vi "6.5test.vi"() -> ()   [LabVIEW 2018]
uses:
  <vilib>/Instr/_visa.llb/VISA Configure Serial Port (Instr).vi
panel:
  in  "TCP HEX":bool
  in  "设置端口号":string
  in  "创建8266服务器":bool
  in  "字符串3":string
  in  "确定按钮3":bool
  in  "字符串2":string
  in  "确定按钮2":bool
  in  "字符串1":string
  in  "确定按钮1":bool
  in  "多条串口发送":bool
  in  "确定按钮0":bool
  in  "字符串0":string
  in  "清空TCP内容":bool
  in  "TCP发送消息框":string
  in  "TCP发送":bool
  in  "服务器发送":bool
  in  "远程端口":u16
  in  "远程IP":string
  in  "开启监听":bool
  in  "查看当前建立连接":bool
  out "TCP接收信息框":string
  in  "自动添加回车":bool
  in  "十六进制发送":bool
  in  "串口HEX":bool
  in  "清空数据":bool
  in  "IP按钮":bool
  in  "WIFI密码":string
  in  "WIFI用户名":string
  in  "连入wifi":bool
  in  "重启按钮":bool
  in  "AT测试按钮":bool
  in  "停止":bool
  out "串口接收信息框":string
  in  "串口发送":bool
  in  "串口发送消息框":string
  in  "baud rate (9600)":u32=9600 caption="波特率"
  in  "VISA resource name":refnum<visa-resource-name> caption="串口号"
  # "串口配置"
  # "TCP CLIENT配置"
  # "ESP8266 功能选择"
  # "串口信息"
  # "TCP CLIENT信息"
  # "多条串口发送 / AT指令"
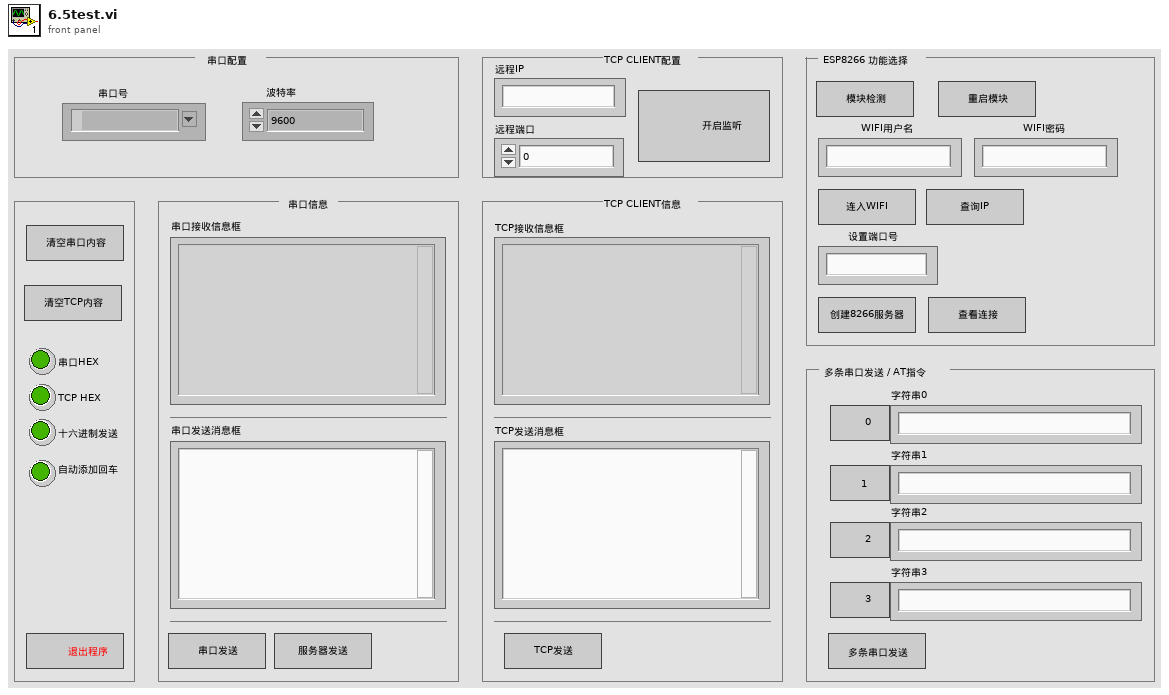
[diagram p1: front panel]
types:
  T1 = enum16{"Standard", "Buffered", "CRLF", "Immediate"}
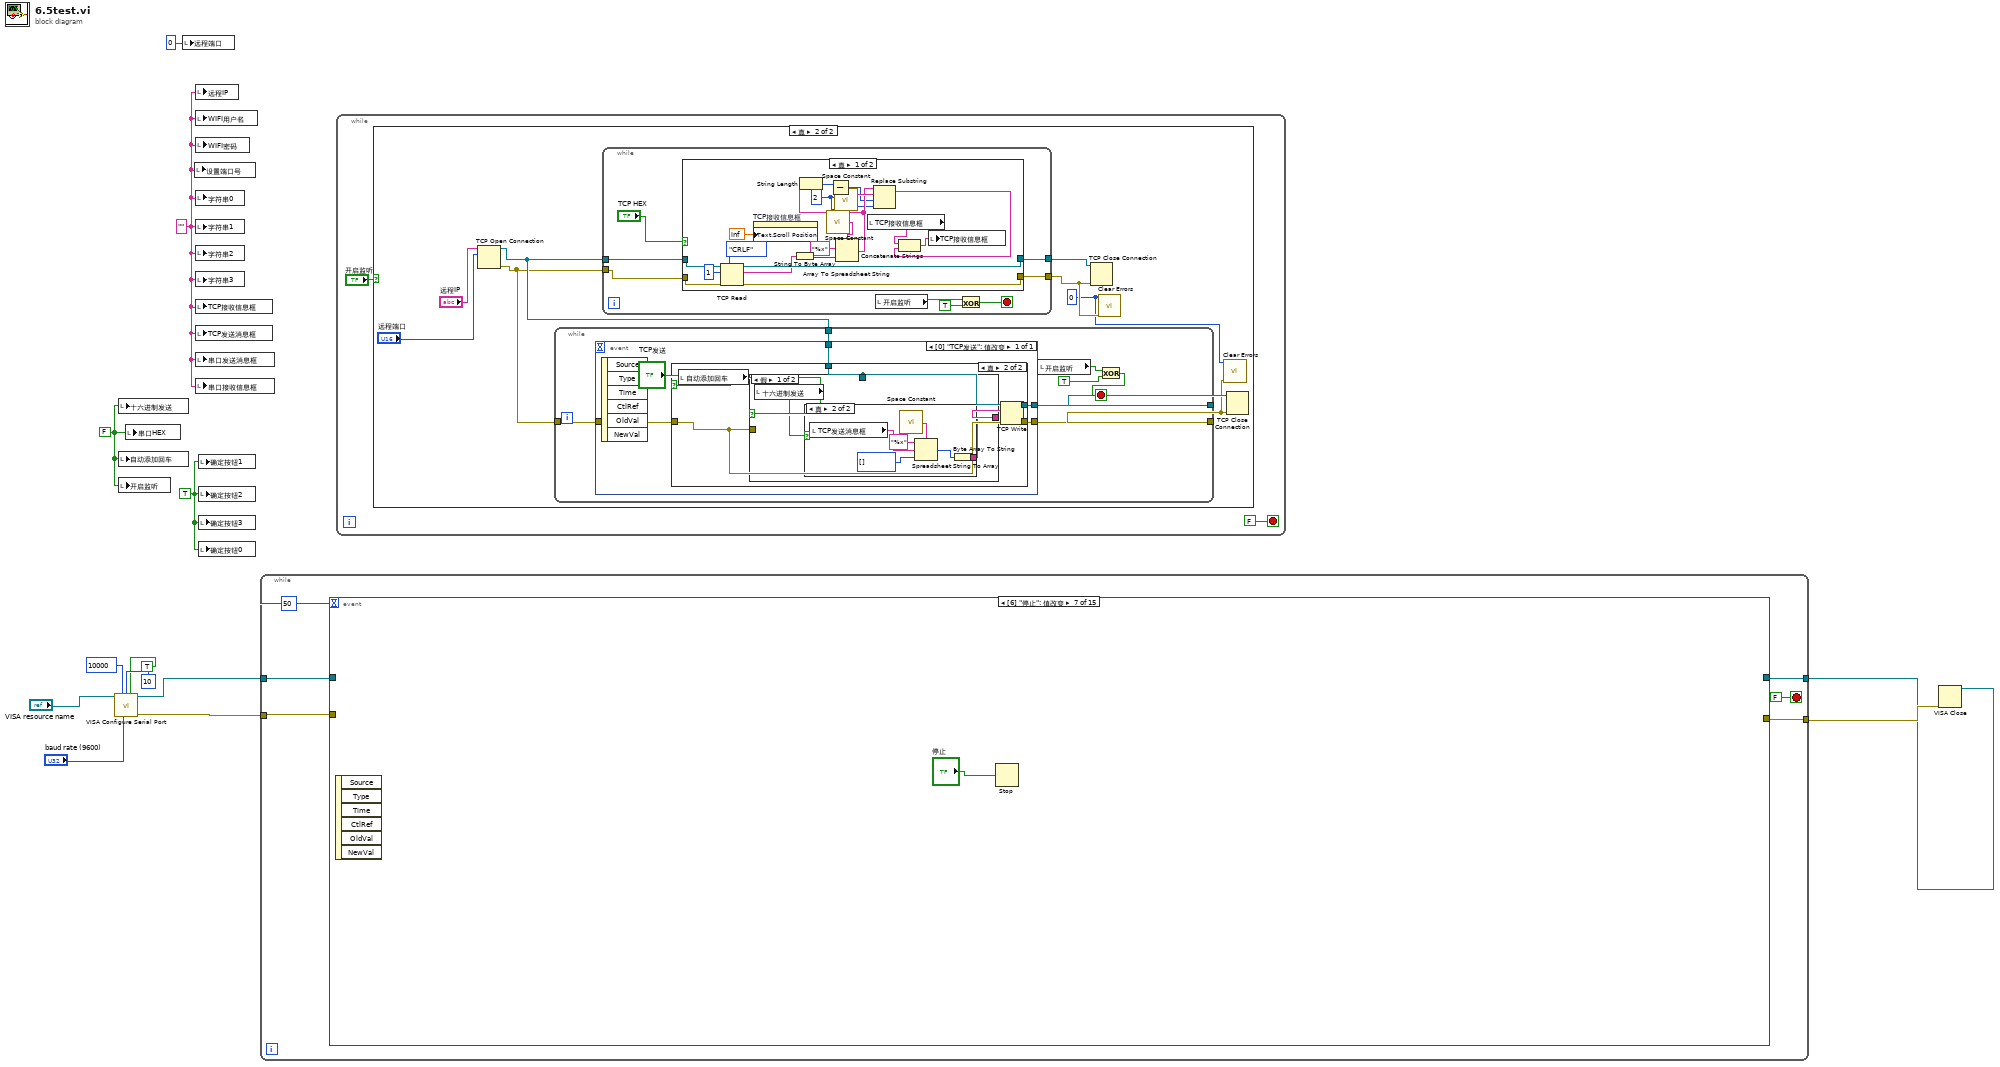
[diagram p0: block diagram]
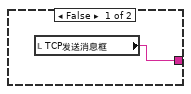
[diagram p4: hidden frame]
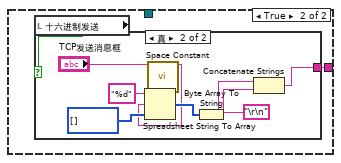
[diagram p5: hidden frame]
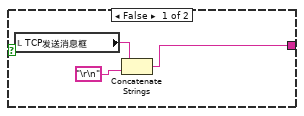
[diagram p6: hidden frame]
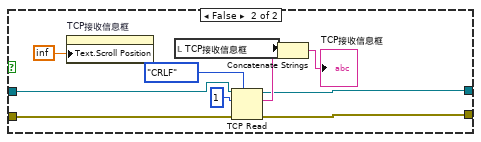
[diagram p7: hidden frame]
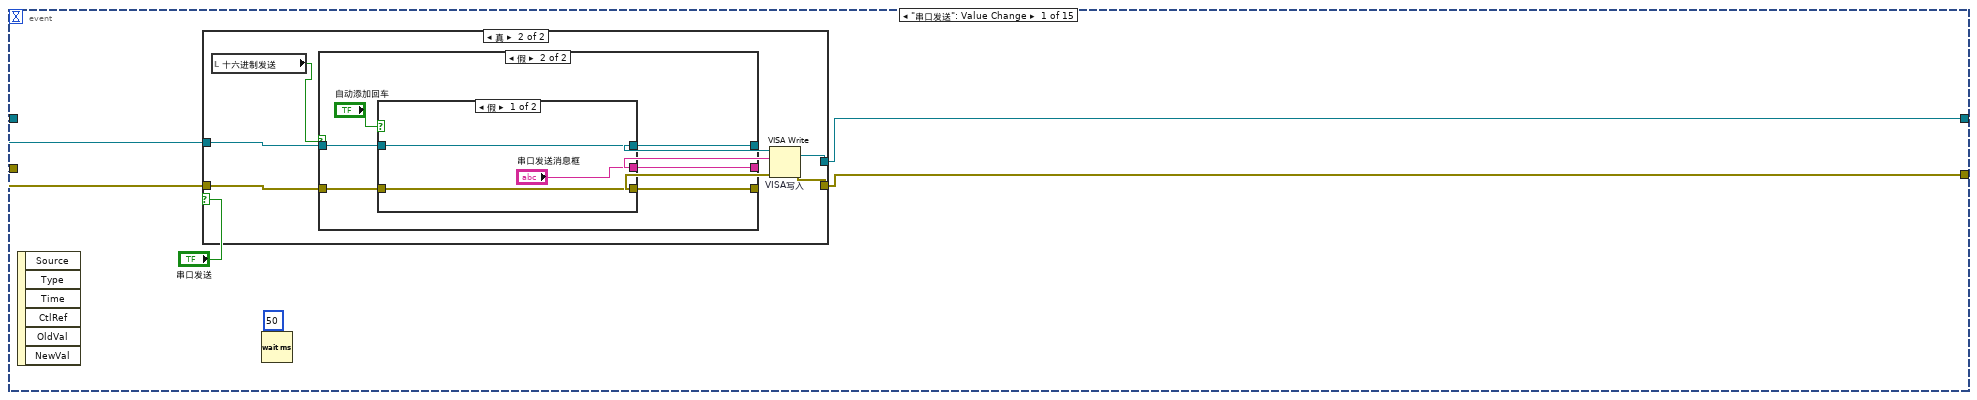
[diagram p8: hidden frame]
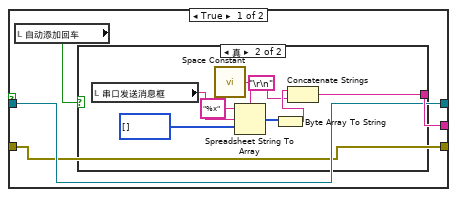
[diagram p10: hidden frame]
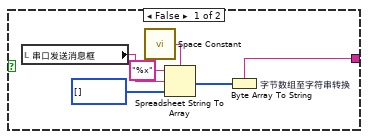
[diagram p11: hidden frame]
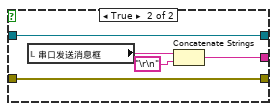
[diagram p12: hidden frame]
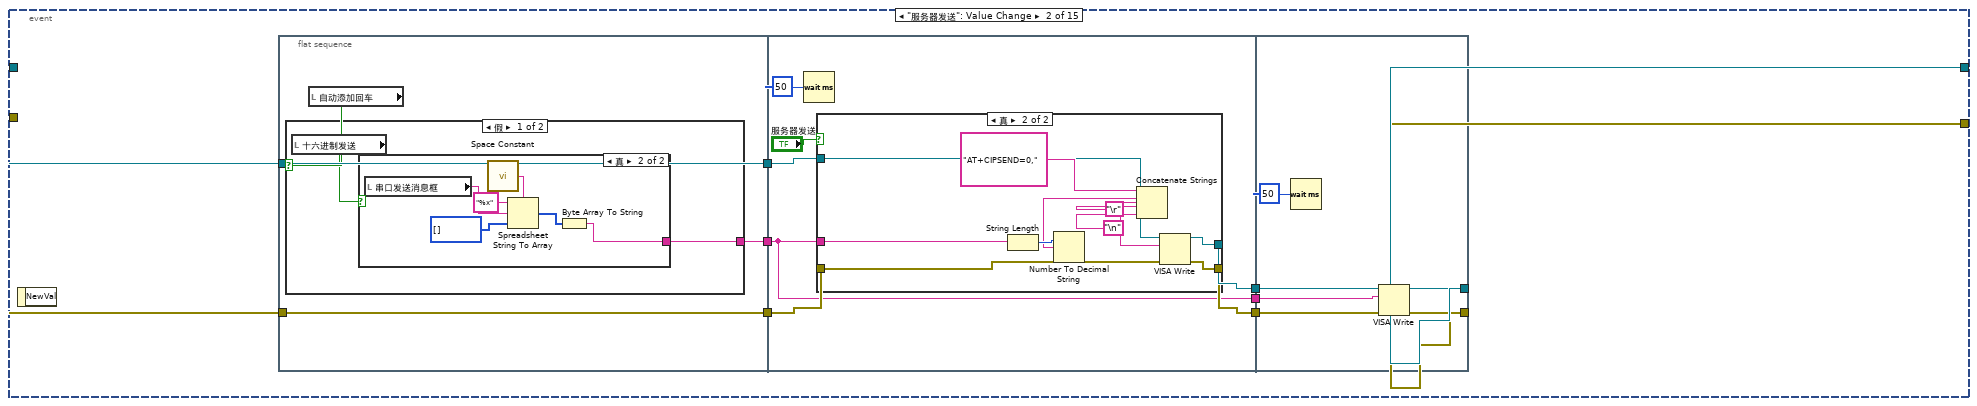
[diagram p13: hidden frame]
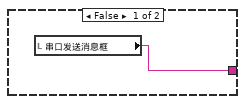
[diagram p14: hidden frame]
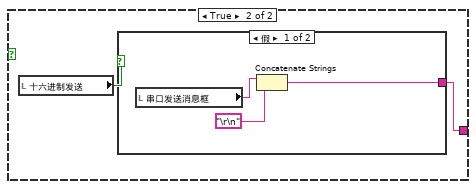
[diagram p15: hidden frame]
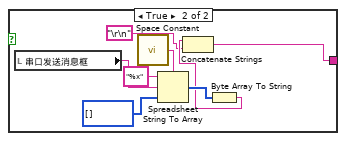
[diagram p16: hidden frame]
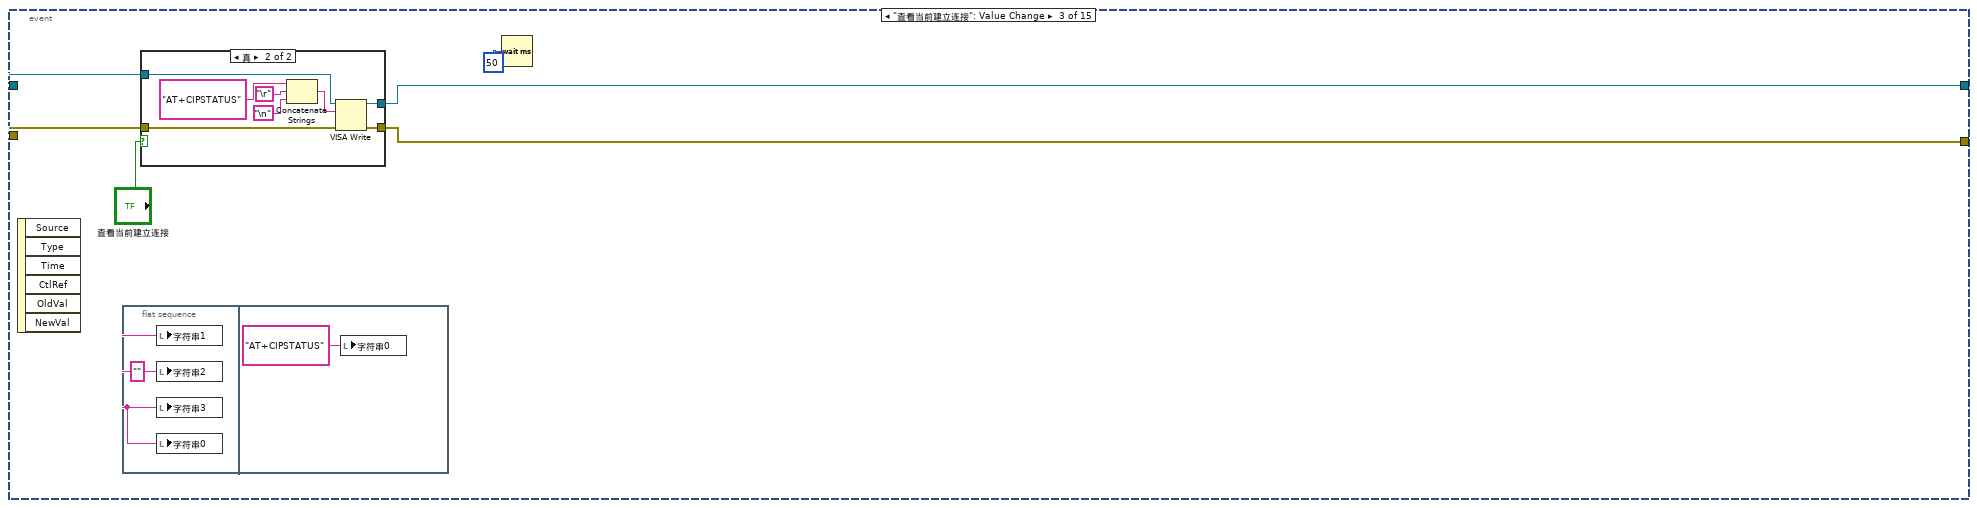
[diagram p18: hidden frame]
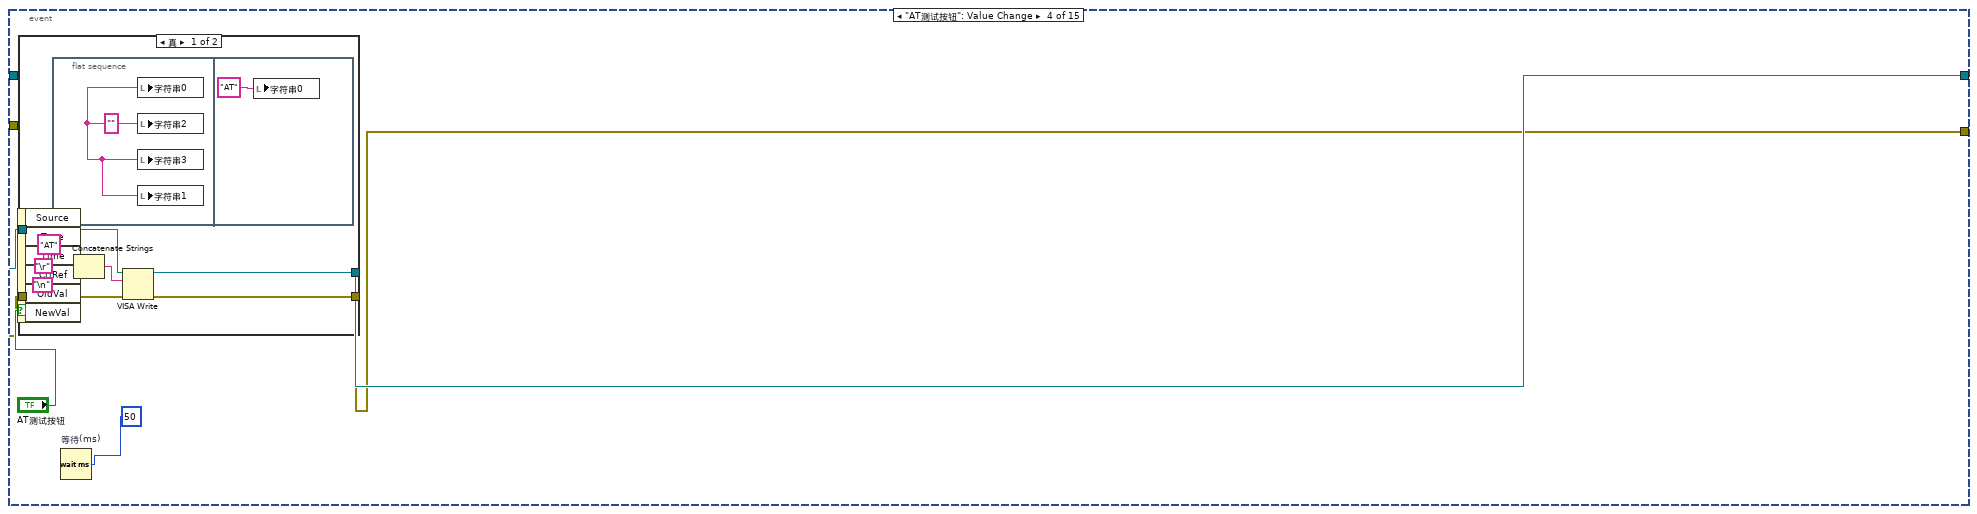
[diagram p20: hidden frame]
diagram:
  w1 = FALSE ("开启监听")
  w2 = "" ("字符串2")
  w4 = TRUE ("确定按钮0")
  n1 = call-poly "VISA Configure Serial Port"("VISA resource name"="VISA resource name", "timeout (10sec)"=u32 10000, "termination char\n(0xA = '\\n' = LF)"=u8 10 ("termination char\n(0xA = '\\n' = LF)"), "Enable Termination\nChar (T)"=TRUE ("Enable Termination\nChar (T)"), "baud rate (9600)"="baud rate (9600)") -> ("VISA resource name out"=w7:refnum<visa-resource-name>, "error out"=w6:errorcluster)  [unwired: 9 in]
  n2 = local write "十六进制发送"(w1) -> ()
  n3 = local write "自动添加回车"(w1) -> ()
  n4 = local write "开启监听"(w1) -> ()
  n5 = local write "串口HEX"(w1) -> ()
  n6 = local write "远程端口"(u16 0 ("远程端口")) -> ()
  n7 = local write "设置端口号"(w2) -> ()
  n8 = local write "远程IP"(w2) -> ()
  n9 = local write "WIFI用户名"(w2) -> ()
  n10 = local write "WIFI密码"(w2) -> ()
  n11 = local write "字符串0"(w2) -> ()
  n12 = local write "字符串1"(w2) -> ()
  n13 = local write "字符串2"(w2) -> ()
  n14 = local write "字符串3"(w2) -> ()
  n15 = local write "TCP接收信息框"(w2) -> ()
  n16 = local write "TCP发送消息框"(w2) -> ()
  n17 = local write "串口发送消息框"(w2) -> ()
  n18 = local write "串口接收信息框"(w2) -> ()
  n19 = local write "确定按钮1"(w4) -> ()
  n20 = local write "确定按钮2"(w4) -> ()
  n21 = local write "确定按钮3"(w4) -> ()
  n22 = local write "确定按钮0"(w4) -> ()
  n23 = while {
    tunnel: w6 -> [w18]
    tunnel: w7 -> [w19]
    tunnel: [w15] -> w5
    tunnel: [w14] -> w8
    stop <- FALSE stop-if-true
    n24 = event shown="[6] \"停止\": 值改变" {
      selector: _ -> [_ _ _ _ _ _ _ _ _ _ _ _ _ _ _]
      dyn-events: _ -> [_ _ _ _ _ _ _ _ _ _ _ _ _ _ _]
      timeout: 50 -> [_ _ _ _ _ _ _ _ _ _ _ _ _ _ _]
      tunnel: w19 -> [w24 w77 w132 w148 w172 w197 _ w214 w237 w301 w388 _ _ _ _]
      tunnel: w18 -> [w23 w76 w131 w147 w171 w196 _ w213 w236 w300 w387 _ _ _ _]
      tunnel: [w22 w73 w130 w146 w170 w195 _ w212 w235 w298 w386 _ _ _ _] -> w15
      tunnel: [w21 w72 w129 w145 w169 w194 _ w211 w234 w299 w385 _ _ _ _] -> w14
      event "串口发送": Value Change {
        n25 = event-data() -> ()  [unwired: 1 in, 6 out]
        n26 = case shown="真" "串口发送" {
          tunnel: w24 -> [w27 w35]
          tunnel: w23 -> [w26 w34]
          tunnel: [w27 w31] -> w22
          tunnel: [w26 w32] -> w21
          frame False {
          }
          frame True {
            n27 = local read "十六进制发送"() -> (w28:bool)
            n28 = case shown="假" w28 {
              tunnel: w35 -> [w38 w59]
              tunnel: w34 -> [w37 w58]
              tunnel: [w39 w57] -> w33
              tunnel: [w38 w55] -> w30
              tunnel: [w37 w54] -> w29
              frame True {
                n29 = local read "自动添加回车"() -> (w36:bool)
                n30 = case shown="真" w36 {
                  tunnel: [w40 w47] -> w39
                  frame False {
                    n31 = local read "串口发送消息框"() -> (w44:string)
                    n32 = call <vilib>:"Space Constant.vi"() -> ("String"=w45:string)
                    n33 = Spreadsheet String To Array(delimiter (Tab)=w45, format string="%x" ("格式字符串"), spreadsheet string=w44, array type (2D Dbl)=u8[] []) -> (array=w41:u8[])
                    n34 = Byte Array To String "字节数组至字符串转换"(unsigned byte array=w41) -> (string=w40:string)
                  }
                  frame True {
                    n35 = local read "串口发送消息框"() -> (w51:string)
                    n36 = call <vilib>:"Space Constant.vi"() -> ("String"=w52:string)
                    n37 = Spreadsheet String To Array(delimiter (Tab)=w52, format string="%x" ("格式字符串"), spreadsheet string=w51, array type (2D Dbl)=u8[] []) -> (array=w53:u8[])
                    n38 = Byte Array To String(unsigned byte array=w53) -> (string=w48:string)
                    n39 = Concatenate Strings(w48, "\r\n") -> (w47:string)
                  }
                }
              }
              frame False {
                n40 = case shown="假" "自动添加回车" {
                  tunnel: w59 -> [w61 w66]
                  tunnel: w58 -> [w60 w65]
                  tunnel: ["串口发送消息框" w67] -> w57
                  tunnel: [w61 w66] -> w55
                  tunnel: [w60 w65] -> w54
                  frame False {
                  }
                  frame True {
                    n41 = local read "串口发送消息框"() -> (w63:string)
                    n42 = Concatenate Strings ("连接字符串")(w63, "\r\n") -> (w67:string)
                  }
                }
              }
            }
            n43 = VISA Write "VISA写入"(VISA resource name=w30, write buffer=w33, error in (no error)=w29) -> (VISA resource name out=w31:refnum<visa-resource-name>, error out=w32:errorcluster)  [unwired: 1 out]
          }
        }
        n44 = Wait (ms)(milliseconds to wait=u32 50 ("等待时间（毫秒）")) -> ()  [unwired: 1 out]
      }
      event "服务器发送": Value Change {
        n45 = event-data() -> ()  [unwired: 1 in, 1 out]
        n46 = flat-sequence {
          tunnel: w76 -> [w80]
          tunnel: w77 -> [w81]
          tunnel: [w81] -> w71
          tunnel: [w80] -> w70
          tunnel: [w78] -> w69
          tunnel: [w107] -> w75
          tunnel: [w106] -> w74
          tunnel: w71 -> [w109]
          tunnel: w70 -> [w108]
          tunnel: w69 -> [w104]
          tunnel: [w104] -> w68
          tunnel: w75 -> [w127]
          tunnel: w74 -> [w126]
          tunnel: [w124] -> w73
          tunnel: [w123] -> w72
          tunnel: w68 -> [w122]
          frame #0 {
            n47 = local read "自动添加回车"() -> (w79:bool)
            n48 = case shown="假" w79 {
              tunnel: [w82 w91] -> w78
              frame False {
                n49 = local read "十六进制发送"() -> (w83:bool)
                n50 = case shown="真" w83 {
                  tunnel: [w84 w85] -> w82
                  frame False {
                    n51 = local read "串口发送消息框"() -> (w84:string)
                  }
                  frame True {
                    n52 = local read "串口发送消息框"() -> (w90:string)
                    n53 = call <vilib>:"Space Constant.vi"() -> ("String"=w89:string)
                    n54 = Spreadsheet String To Array(delimiter (Tab)=w89, format string="%x" ("格式字符串"), spreadsheet string=w90, array type (2D Dbl)=u8[] []) -> (array=w88:u8[])
                    n55 = Byte Array To String(unsigned byte array=w88) -> (string=w85:string)
                  }
                }
              }
              frame True {
                n56 = local read "十六进制发送"() -> (w92:bool)
                n57 = case shown="假" w92 {
                  tunnel: [w93 w96] -> w91
                  frame False {
                    n58 = local read "串口发送消息框"() -> (w95:string)
                    n59 = Concatenate Strings(w95, "\r\n") -> (w93:string)
                  }
                  frame True {
                    n60 = local read "串口发送消息框"() -> (w101:string)
                    n61 = call <vilib>:"Space Constant.vi"() -> ("String"=w102:string)
                    n62 = Spreadsheet String To Array(delimiter (Tab)=w102, format string="%x" ("格式字符串"), spreadsheet string=w101, array type (2D Dbl)=u8[] []) -> (array=w103:u8[])
                    n63 = Byte Array To String(unsigned byte array=w103) -> (string=w98:string)
                    n64 = Concatenate Strings(w98, "\r\n") -> (w96:string)
                  }
                }
              }
            }
          }
          frame #1 {
            n65 = Wait (ms)(milliseconds to wait=u32 50 ("等待时间（毫秒）")) -> ()  [unwired: 1 out]
            n66 = case shown="真" "服务器发送" {
              tunnel: w109 -> [_ w117]
              tunnel: w108 -> [_ w116]
              tunnel: [_ w115] -> w107
              tunnel: [_ w114] -> w106
              tunnel: w104 -> [_ w111]
              frame False {
              }
              frame True {
                n67 = String Length(string=w111) -> (length=w113:i32)
                n68 = Number To Decimal String(number=w113) -> (decimal integer string=w112:string)  [unwired: 1 in]
                n69 = Concatenate Strings("AT+CIPSEND=0," ("字符串"), w112, "\r", "\n") -> (w118:string)
                n70 = VISA Write ("VISA写入")(VISA resource name=w117, write buffer=w118, error in (no error)=w116) -> (VISA resource name out=w115:refnum<visa-resource-name>, error out=w114:errorcluster)  [unwired: 1 out]
              }
            }
          }
          frame #2 {
            n71 = Wait (ms)(milliseconds to wait=u32 50 ("等待时间（毫秒）")) -> ()  [unwired: 1 out]
            n72 = VISA Write(VISA resource name=w127, write buffer=w122, error in (no error)=w126) -> (VISA resource name out=w124:refnum<visa-resource-name>, error out=w123:errorcluster)  [unwired: 1 out]
          }
        }
      }
      event "查看当前建立连接": Value Change {
        n73 = event-data() -> ()  [unwired: 1 in, 6 out]
        n74 = flat-sequence {
          frame #0 {
            w134 = "" ("字符串0")
            n75 = local write "字符串1"(w134) -> ()
            n76 = local write "字符串2"(w134) -> ()
            n77 = local write "字符串3"(w134) -> ()
            n78 = local write "字符串0"(w134) -> ()
          }
          frame #1 {
            n79 = local write "字符串0"("AT+CIPSTATUS" ("字符串")) -> ()
          }
        }
        n80 = case shown="真" "查看当前建立连接" {
          tunnel: w132 -> [_ w139]
          tunnel: w131 -> [_ w138]
          tunnel: [_ w137] -> w130
          tunnel: [_ w136] -> w129
          frame False {
          }
          frame True {
            n81 = Concatenate Strings("AT+CIPSTATUS" ("字符串"), "\r", "\n") -> (w140:string)
            n82 = VISA Write ("VISA写入")(VISA resource name=w139, write buffer=w140, error in (no error)=w138) -> (VISA resource name out=w137:refnum<visa-resource-name>, error out=w136:errorcluster)  [unwired: 1 out]
          }
        }
        n83 = Wait (ms)(milliseconds to wait=u32 50 ("等待时间（毫秒）")) -> ()  [unwired: 1 out]
      }
      event "AT测试按钮": Value Change {
        n84 = event-data() -> ()  [unwired: 1 in, 6 out]
        n85 = case shown="真" "AT测试按钮" {
          tunnel: w148 -> [w157 w167]
          tunnel: w147 -> [w156 w166]
          tunnel: [w155 w165] -> w146
          tunnel: [w154 w164] -> w145
          frame True {
            n86 = flat-sequence {
              frame #0 {
                w158 = "" ("字符串1")
                n87 = local write "字符串0"(w158) -> ()
                n88 = local write "字符串2"(w158) -> ()
                n89 = local write "字符串3"(w158) -> ()
                n90 = local write "字符串1"(w158) -> ()
              }
              frame #1 {
                n91 = local write "字符串0"("AT" ("字符串")) -> ()
              }
            }
            n92 = Concatenate Strings("AT" ("字符串"), "\r", "\n") -> (w150:string)
            n93 = VISA Write(VISA resource name=w157, write buffer=w150, error in (no error)=w156) -> (VISA resource name out=w155:refnum<visa-resource-name>, error out=w154:errorcluster)  [unwired: 1 out]
          }
          frame False {
            n94 = Concatenate Strings("AT" ("字符串"), "\r", "\n") -> (w160:string)
            n95 = VISA Write(VISA resource name=w167, write buffer=w160, error in (no error)=w166) -> (VISA resource name out=w165:refnum<visa-resource-name>, error out=w164:errorcluster)  [unwired: 1 out]
          }
        }
        n96 = Wait (ms) "等待(ms)"(milliseconds to wait=u32 50 ("等待时间（毫秒）")) -> ()  [unwired: 1 out]
      }
      event "连入wifi": Value Change {
        n97 = event-data() -> ()  [unwired: 1 in, 6 out]
        n98 = flat-sequence {
          frame #0 {
            w174 = "" ("字符串0")
            n99 = local write "字符串1"(w174) -> ()
            n100 = local write "字符串2"(w174) -> ()
            n101 = local write "字符串3"(w174) -> ()
            n102 = local write "字符串0"(w174) -> ()
          }
          frame #1 {
            n103 = local read "WIFI用户名"() -> (w177:string)
            n104 = local read "WIFI密码"() -> (w176:string)
            n105 = Concatenate Strings("AT+CWJAP=\"" ("字符串"), w177, "\",\"" ("字符串"), w176, "\"" ("字符串")) -> (w175:string)
            n106 = local write "字符串0"(w175) -> ()
          }
        }
        n107 = case shown="真" "连入wifi" {
          tunnel: w172 -> [_ w184]
          tunnel: w171 -> [_ w183]
          tunnel: [_ w182] -> w170
          tunnel: [_ w181] -> w169
          frame False {
          }
          frame True {
            n108 = Concatenate Strings("AT+CWJAP=\"" ("字符串"), "WIFI用户名", "\",\"" ("字符串"), "WIFI密码", "\"" ("字符串"), "\r", "\n") -> (w191:string)
            n109 = VISA Write(VISA resource name=w184, write buffer=w191, error in (no error)=w183) -> (VISA resource name out=w182:refnum<visa-resource-name>, error out=w181:errorcluster)  [unwired: 1 out]
          }
        }
        n110 = Wait (ms)(milliseconds to wait=u32 50 ("等待时间（毫秒）")) -> ()  [unwired: 1 out]
      }
      event "IP按钮": Value Change {
        n111 = event-data() -> ()  [unwired: 1 in, 6 out]
        n112 = Wait (ms)(milliseconds to wait=u32 50 ("等待时间（毫秒）")) -> ()  [unwired: 1 out]
        n113 = case shown="真" "IP按钮" {
          tunnel: w197 -> [_ w204]
          tunnel: w196 -> [_ w203]
          tunnel: [_ w202] -> w195
          tunnel: [_ w201] -> w194
          frame False {
          }
          frame True {
            n114 = Concatenate Strings("AT+CIPSTA?" ("字符串"), "\r", "\n") -> (w205:string)
            n115 = VISA Write(VISA resource name=w204, write buffer=w205, error in (no error)=w203) -> (VISA resource name out=w202:refnum<visa-resource-name>, error out=w201:errorcluster)  [unwired: 1 out]
          }
        }
        n116 = flat-sequence {
          frame #0 {
            w199 = "" ("字符串1")
            n117 = local write "字符串0"(w199) -> ()
            n118 = local write "字符串2"(w199) -> ()
            n119 = local write "字符串3"(w199) -> ()
            n120 = local write "字符串1"(w199) -> ()
          }
          frame #1 {
            n121 = local write "字符串0"("AT+CIPSTA?" ("字符串")) -> ()
          }
        }
      }
      event "停止": Value Change {
        n122 = event-data() -> ()  [unwired: 1 in, 6 out]
        n123 = Stop(stop? (T)="停止") -> ()
      }
      event "重启按钮": Value Change {
        n124 = event-data() -> ()  [unwired: 1 in, 6 out]
        n125 = case shown="真" "重启按钮" {
          tunnel: w214 -> [w221 w229]
          tunnel: w213 -> [w220 w228]
          tunnel: [w219 w227] -> w212
          tunnel: [w218 w226] -> w211
          frame True {
            n126 = Concatenate Strings("AT+RST" ("字符串"), "\r", "\n") -> (w222:string)
            n127 = VISA Write(VISA resource name=w221, write buffer=w222, error in (no error)=w220) -> (VISA resource name out=w219:refnum<visa-resource-name>, error out=w218:errorcluster)  [unwired: 1 out]
          }
          frame False {
            n128 = Concatenate Strings("AT+RST" ("字符串"), "\r", "\n") -> (w230:string)
            n129 = VISA Write(VISA resource name=w229, write buffer=w230, error in (no error)=w228) -> (VISA resource name out=w227:refnum<visa-resource-name>, error out=w226:errorcluster)  [unwired: 1 out]
          }
        }
        n130 = Wait (ms)(milliseconds to wait=u32 50 ("等待时间（毫秒）")) -> ()  [unwired: 1 out]
        n131 = flat-sequence {
          frame #0 {
            w216 = "" ("字符串1")
            n132 = local write "字符串0"(w216) -> ()
            n133 = local write "字符串2"(w216) -> ()
            n134 = local write "字符串3"(w216) -> ()
            n135 = local write "字符串1"(w216) -> ()
          }
          frame #1 {
            n136 = local write "字符串0"("AT+RST" ("字符串")) -> ()
          }
        }
      }
      event Timeout {
        n137 = event-data() -> ()  [unwired: 1 in, 3 out]
        n138 = property class="Instr"(reference=w237, error in=w236) -> (reference out=w238:refnum<visa-resource-name>, error out=w239:errorcluster, "Bytes at Port"=w241:u32)
        n139 = Not Equal To 0?(x=w241) -> (x != 0?=w240:bool)
        n140 = case shown="真" w240 {
          tunnel: [_ w247] -> w235
          tunnel: [_ w246] -> w234
          tunnel: w238 -> [_ w245]
          tunnel: w239 -> [_ w244]
          tunnel: w241 -> [_ w243]
          frame False {
          }
          frame True {
            n141 = case shown="真" "串口HEX" {
              tunnel: [_ w297] -> w247
              tunnel: w245 -> [_ w296]
              tunnel: w244 -> [_ w295]
              tunnel: w243 -> [_ w294]
              tunnel: [_ w291] -> w246
              tunnel: w244 -> [w253 _]
              tunnel: w243 -> [w252 _]
              tunnel: w245 -> [w251 _]
              tunnel: w245 -> [w250 _]
              tunnel: w244 -> [w249 _]
              tunnel: w243 -> [w248 _]
              frame True {
                n142 = local read "TCP发送消息框"() -> (w256:string)
                n143 = String Length(string=w256) -> (length=w255:i32)
                n144 = Equal To 0?(x=w255) -> (x = 0?=w254:bool)
                n145 = case shown="假" w254 {
                  tunnel: w253 -> [_ w275]
                  tunnel: w252 -> [_ w274]
                  tunnel: w251 -> [_ w273]
                  tunnel: [w258 w272] -> _
                  tunnel: [w259 w270] -> _
                  tunnel: w250 -> [w262 _]
                  tunnel: w249 -> [w261 _]
                  tunnel: w248 -> [w257 _]
                  frame False {
                    n146 = VISA Read(VISA resource name=w262, byte count=w257, error in (no error)=w261) -> (VISA resource name out=w259:refnum<visa-resource-name>, read buffer=w260:string, error out=w258:errorcluster)  [unwired: 1 out]
                    n147 = local read "串口接收信息框"() -> (w264:string)
                    n148 = String To Byte Array(string=w260) -> (unsigned byte array=w268:u8[])
                    n149 = call <vilib>:"Space Constant.vi"() -> ("String"=w266:string)
                    n150 = property on="串口接收信息框" class="Str"("Text.Scroll Position"=inf) -> ()  [unwired: 2 in, 2 out]
                    n151 = Array To Spreadsheet String(delimiter (Tab)=w266, array=w268, 3:"%x" ("格式字符串")) -> (spreadsheet string=w265:string)
                    n152 = Concatenate Strings(w264, w265) -> (w263:string)
                    n153 = local write "串口接收信息框"(w263) -> ()
                  }
                  frame True {
                    n154 = VISA Read(VISA resource name=w273, byte count=w274, error in (no error)=w275) -> (VISA resource name out=w270:refnum<visa-resource-name>, read buffer=w271:string, error out=w272:errorcluster)  [unwired: 1 out]
                    n155 = local read "串口接收信息框"() -> (w285:string)
                    n156 = String To Byte Array(string=w271) -> (unsigned byte array=w288:u8[])
                    n157 = property on="串口接收信息框" class="Str"("Text.Scroll Position"=inf) -> ()  [unwired: 2 in, 2 out]
                    n158 = call <vilib>:"Space Constant.vi"() -> ("String"=w286:string)
                    n159 = Array To Spreadsheet String(delimiter (Tab)=w286, array=w288, 3:"%x" ("格式字符串")) -> (spreadsheet string=w278:string)
                    n160 = String Length(string=w278) -> (length=w282:i32)
                    n161 = call <vilib>:"Space Constant.vi"() -> ("String"=w276:string)
                    n162 = Subtract(x=w282, y=2) -> (x-y=w280:i32)
                    n163 = Replace Substring(2:2 ("长度（子字符串长度）"), 3:w280, 4:w276, 5:w278) -> (1:w277:string)  [unwired: 1 out]
                    n164 = Concatenate Strings(w285, w277) -> (w284:string)
                    n165 = local write "串口接收信息框"(w284) -> ()
                  }
                }
              }
              frame False {
                n166 = local read "串口接收信息框"() -> (w293:string)
                n167 = property on="串口接收信息框" class="Str"("Text.Scroll Position"=inf) -> ()  [unwired: 2 in, 2 out]
                n168 = VISA Read(VISA resource name=w296, byte count=w294, error in (no error)=w295) -> (VISA resource name out=w297:refnum<visa-resource-name>, read buffer=w290:string, error out=w291:errorcluster)  [unwired: 1 out]
                n169 = Concatenate Strings(w293, w290) -> (→"串口接收信息框":string)
              }
            }
          }
        }
      }
      event "多条串口发送": Value Change {
        n170 = event-data() -> ()  [unwired: 1 in, 6 out]
        n171 = case shown="真" "多条串口发送" {
          tunnel: w301 -> [_ w312]
          tunnel: w300 -> [_ w311]
          tunnel: [_ w308] -> w298
          tunnel: [_ w307] -> w299
          frame False {
          }
          frame True {
            n172 = flat-sequence {
              tunnel: w312 -> [w317]
              tunnel: w311 -> [w316]
              tunnel: [w315] -> w310
              tunnel: [w314] -> w309
              tunnel: w310 -> [w334]
              tunnel: w309 -> [w333]
              tunnel: [w332] -> w306
              tunnel: [w331] -> w305
              tunnel: w306 -> [w352]
              tunnel: w305 -> [w351]
              tunnel: [w350] -> w304
              tunnel: [w349] -> w303
              tunnel: [w367] -> w307
              tunnel: [w368] -> w308
              tunnel: w304 -> [w370]
              tunnel: w303 -> [w369]
              frame #0 {
                n173 = case shown="真" "确定按钮0" {
                  tunnel: w317 -> [w320 w326]
                  tunnel: w316 -> [w319 w325]
                  tunnel: [w320 w322] -> w315
                  tunnel: [w319 w321] -> w314
                  frame False {
                  }
                  frame True {
                    n174 = local read "自动添加回车"() -> (w324:bool)
                    n175 = case shown="真" w324 {
                      tunnel: [w327 w328] -> w323
                      frame False {
                        n176 = local read "字符串0"() -> (w327:string)
                      }
                      frame True {
                        n177 = Concatenate Strings("字符串0", "\r\n") -> (w328:string)
                      }
                    }
                    n178 = VISA Write(VISA resource name=w326, write buffer=w323, error in (no error)=w325) -> (VISA resource name out=w322:refnum<visa-resource-name>, error out=w321:errorcluster)  [unwired: 1 out]
                  }
                }
                n179 = Wait (ms)(milliseconds to wait=u32 50 ("等待时间（毫秒）")) -> ()  [unwired: 1 out]
              }
              frame #1 {
                n180 = case shown="真" "确定按钮1" {
                  tunnel: w334 -> [w338 w344]
                  tunnel: w333 -> [w337 w343]
                  tunnel: [w338 w340] -> w332
                  tunnel: [w337 w339] -> w331
                  frame False {
                  }
                  frame True {
                    n181 = local read "自动添加回车"() -> (w342:bool)
                    n182 = case shown="假" w342 {
                      tunnel: [w345 w346] -> w341
                      frame False {
                        n183 = local read "字符串1"() -> (w345:string)
                      }
                      frame True {
                        n184 = Concatenate Strings("字符串1", "\r\n") -> (w346:string)
                      }
                    }
                    n185 = VISA Write(VISA resource name=w344, write buffer=w341, error in (no error)=w343) -> (VISA resource name out=w340:refnum<visa-resource-name>, error out=w339:errorcluster)  [unwired: 1 out]
                  }
                }
                n186 = Wait (ms)(milliseconds to wait=u32 50 ("等待时间（毫秒）")) -> ()  [unwired: 1 out]
              }
              frame #2 {
                n187 = case shown="真" "确定按钮2" {
                  tunnel: w352 -> [w356 w362]
                  tunnel: w351 -> [w355 w361]
                  tunnel: [w356 w358] -> w350
                  tunnel: [w355 w357] -> w349
                  frame False {
                  }
                  frame True {
                    n188 = local read "自动添加回车"() -> (w360:bool)
                    n189 = case shown="假" w360 {
                      tunnel: [w363 w364] -> w359
                      frame False {
                        n190 = local read "字符串2"() -> (w363:string)
                      }
                      frame True {
                        n191 = Concatenate Strings("字符串2", "\r\n") -> (w364:string)
                      }
                    }
                    n192 = VISA Write(VISA resource name=w362, write buffer=w359, error in (no error)=w361) -> (VISA resource name out=w358:refnum<visa-resource-name>, error out=w357:errorcluster)  [unwired: 1 out]
                  }
                }
                n193 = Wait (ms)(milliseconds to wait=u32 50 ("等待时间（毫秒）")) -> ()  [unwired: 1 out]
              }
              frame #3 {
                n194 = case shown="真" "确定按钮3" {
                  tunnel: w370 -> [w374 w380]
                  tunnel: w369 -> [w373 w379]
                  tunnel: [w374 w376] -> w368
                  tunnel: [w373 w375] -> w367
                  frame False {
                  }
                  frame True {
                    n195 = local read "自动添加回车"() -> (w378:bool)
                    n196 = case shown="假" w378 {
                      tunnel: [w381 w382] -> w377
                      frame False {
                        n197 = local read "字符串3"() -> (w381:string)
                      }
                      frame True {
                        n198 = Concatenate Strings("字符串3", "\r\n") -> (w382:string)
                      }
                    }
                    n199 = VISA Write(VISA resource name=w380, write buffer=w377, error in (no error)=w379) -> (VISA resource name out=w376:refnum<visa-resource-name>, error out=w375:errorcluster)  [unwired: 1 out]
                  }
                }
                n200 = Wait (ms)(milliseconds to wait=u32 50 ("等待时间（毫秒）")) -> ()  [unwired: 1 out]
              }
            }
          }
        }
      }
      event "创建8266服务器": Value Change {
        n201 = event-data() -> ()  [unwired: 1 in, 6 out]
        n202 = case shown="真" "创建8266服务器" {
          tunnel: w388 -> [_ w397]
          tunnel: w387 -> [_ w396]
          tunnel: [_ w391] -> w386
          tunnel: [_ w390] -> w385
          frame False {
          }
          frame True {
            n203 = flat-sequence {
              tunnel: w397 -> [w416]
              tunnel: w396 -> [w415]
              tunnel: [w410] -> w395
              tunnel: [w409] -> w394
              tunnel: w395 -> [w424]
              tunnel: w394 -> [w423]
              tunnel: [w419] -> w393
              tunnel: [w418] -> w392
              tunnel: w393 -> [w433]
              tunnel: w392 -> [w432]
              tunnel: [w431] -> w391
              tunnel: [w430] -> w390
              frame #0 {
                n204 = local write "字符串3"("" ("字符串0")) -> ()
                n205 = local write "字符串2"("" ("字符串0")) -> ()
                n206 = local write "字符串1"("" ("字符串0")) -> ()
                n207 = local write "字符串0"("" ("字符串0")) -> ()
              }
              frame #1 {
                n208 = Concatenate Strings("AT+CIPMUX=1" ("字符串1")) -> (w403:string)
                n209 = Concatenate Strings("AT+CWMODE=3" ("字符串0")) -> (w405:string)
                n210 = Concatenate Strings("AT+CIPSERVER=1,", "设置端口号") -> (w407:string)
                n211 = local write "字符串1"(w403) -> ()
                n212 = local write "字符串0"(w405) -> ()
                n213 = local write "字符串2"(w407) -> ()
              }
              frame #2 {
                n214 = Wait (ms)(milliseconds to wait=u32 50 ("等待时间（毫秒）")) -> ()  [unwired: 1 out]
                n215 = Concatenate Strings("AT+CWMODE=3" ("字符串0"), "\r\n") -> (w412:string)
                n216 = VISA Write(VISA resource name=w416, write buffer=w412, error in (no error)=w415) -> (VISA resource name out=w410:refnum<visa-resource-name>, error out=w409:errorcluster)  [unwired: 1 out]
              }
              frame #3 {
                n217 = Wait (ms)(milliseconds to wait=u32 50 ("等待时间（毫秒）")) -> ()  [unwired: 1 out]
                n218 = Concatenate Strings("AT+CIPMUX=1" ("字符串1"), "\r\n") -> (w420:string)
                n219 = VISA Write(VISA resource name=w424, write buffer=w420, error in (no error)=w423) -> (VISA resource name out=w419:refnum<visa-resource-name>, error out=w418:errorcluster)  [unwired: 1 out]
              }
              frame #4 {
                n220 = Wait (ms)(milliseconds to wait=u32 50 ("等待时间（毫秒）")) -> ()  [unwired: 1 out]
                n221 = local read "设置端口号"() -> (w427:string)
                n222 = Concatenate Strings("AT+CIPSERVER=1,", w427, "\r\n") -> (w425:string)
                n223 = VISA Write(VISA resource name=w433, write buffer=w425, error in (no error)=w432) -> (VISA resource name out=w431:refnum<visa-resource-name>, error out=w430:errorcluster)  [unwired: 1 out]
              }
            }
          }
        }
      }
      event "十六进制发送": Value Change {
        n224 = event-data() -> ()  [unwired: 1 in, 6 out]
        n225 = case shown="假" "十六进制发送" {
          frame False {
            n226 = local read "串口发送消息框"() -> (w450:string)
            n227 = local read "TCP发送消息框"() -> (w435:string)
            n228 = Spreadsheet String To Array(delimiter (Tab)=" " ("分隔符(Tab)"), format string="%d" ("格式字符串"), spreadsheet string=w450, array type (2D Dbl)=string[] []) -> (array=w446:string[])
            n229 = Spreadsheet String To Array(delimiter (Tab)=" " ("分隔符(Tab)"), format string="%d" ("格式字符串"), spreadsheet string=w435, array type (2D Dbl)=string[] []) -> (array=w439:string[])
            n230 = Hexadecimal String To Number(string=w446, default (0uL)=u8 0) -> (number=w445:u8[])  [unwired: 1 in, 1 out]
            n231 = Hexadecimal String To Number(string=w439, default (0uL)=u8 0) -> (number=w440:u8[])  [unwired: 1 in, 1 out]
            n232 = Type Cast(x=w445) -> (*(type *) &x=w443:string)  [unwired: 1 in]
            n233 = Type Cast(x=w440) -> (*(type *) &x=w442:string)  [unwired: 1 in]
            n234 = local write "串口发送消息框"(w443) -> ()
            n235 = local write "TCP发送消息框"(w442) -> ()
          }
          frame True {
            n236 = local read "串口发送消息框"() -> (w460:string)
            n237 = local read "TCP发送消息框"() -> (w451:string)
            n238 = String To Byte Array(string=w460) -> (unsigned byte array=w459:u8[])
            n239 = String To Byte Array(string=w451) -> (unsigned byte array=w452:u8[])
            n240 = Array To Spreadsheet String "数组至电子表格字符串转换"(delimiter (Tab)=" " ("分隔符(Tab)"), array=w459, 3:"%x" ("格式字符串")) -> (spreadsheet string=w456:string)
            n241 = Array To Spreadsheet String "数组至电子表格字符串转换"(delimiter (Tab)=" " ("分隔符(Tab)"), array=w452, 3:"%x" ("格式字符串")) -> (spreadsheet string=w455:string)
            n242 = local write "串口发送消息框"(w456) -> ()
            n243 = local write "TCP发送消息框"(w455) -> ()
          }
        }
      }
      event "清空数据": Value Change {
        n244 = event-data() -> ()  [unwired: 1 in, 6 out]
        n245 = case shown="真" "清空数据" {
          frame False {
          }
          frame True {
            n246 = local write "串口接收信息框"("" ("字符串")) -> ()
          }
        }
      }
      event "清空TCP内容": Value Change {
        n247 = event-data() -> ()  [unwired: 1 in, 6 out]
        n248 = case shown="真" "清空TCP内容" {
          frame False {
          }
          frame True {
            n249 = local write "TCP接收信息框"("" ("TCP接收信息框")) -> ()
          }
        }
      }
      event "串口HEX": Value Change {
        n250 = event-data() -> ()  [unwired: 1 in, 6 out]
      }
    }
  }
  n251 = while {
    stop <- FALSE stop-if-true
    n252 = case shown="真" "开启监听" {
      frame False {
      }
      frame True {
        w467 = 0 ("specific error code to clear (0: all)")
        n253 = TCP Open Connection(address="远程IP", remote port or service name="远程端口") -> (connection ID=w472:refnum<k5>, error out=w471:errorcluster)  [unwired: 3 in]
        n254 = while {
          tunnel: w472 -> [w482]
          tunnel: w471 -> [w481]
          tunnel: [w480] -> w470
          tunnel: [w479] -> w468
          stop <- w476 stop-if-true
          n255 = event shown="[0] \"TCP发送\": 值改变" {
            selector: _ -> [_]
            dyn-events: _ -> [_]
            timeout: _ -> [_]
            tunnel: w482 -> [w486]
            tunnel: w481 -> [w485]
            tunnel: [w484] -> w480
            tunnel: [w483] -> w479
            event "TCP发送": Value Change {
              n256 = event-data() -> ()  [unwired: 1 in, 6 out]
              n257 = case shown="真" "TCP发送" {
                tunnel: w486 -> [_ w493]
                tunnel: w485 -> [_ w492]
                tunnel: [_ w488] -> w484
                tunnel: [_ w489] -> w483
                frame False {
                }
                frame True {
                  n258 = local read "自动添加回车"() -> (w491:bool)
                  n259 = case shown="假" w491 {
                    tunnel: w493 -> [_ _]
                    tunnel: w492 -> [_ _]
                    tunnel: [w494 w503] -> w490
                    frame False {
                      n260 = local read "十六进制发送"() -> (w495:bool)
                      n261 = case shown="真" w495 {
                        tunnel: [w496 w497] -> w494
                        frame False {
                          n262 = local read "TCP发送消息框"() -> (w496:string)
                        }
                        frame True {
                          n263 = local read "TCP发送消息框"() -> (w502:string)
                          n264 = call <vilib>:"Space Constant.vi"() -> ("String"=w501:string)
                          n265 = Spreadsheet String To Array(delimiter (Tab)=w501, format string="%x" ("格式字符串"), spreadsheet string=w502, array type (2D Dbl)=u8[] []) -> (array=w500:u8[])
                          n266 = Byte Array To String(unsigned byte array=w500) -> (string=w497:string)
                        }
                      }
                    }
                    frame True {
                      n267 = local read "十六进制发送"() -> (w504:bool)
                      n268 = case shown="真" w504 {
                        tunnel: [w505 w508] -> w503
                        frame False {
                          n269 = local read "TCP发送消息框"() -> (w507:string)
                          n270 = Concatenate Strings(w507, "\r\n") -> (w505:string)
                        }
                        frame True {
                          n271 = call <vilib>:"Space Constant.vi"() -> ("String"=w514:string)
                          n272 = Spreadsheet String To Array(delimiter (Tab)=w514, format string="%d" ("格式字符串"), spreadsheet string="TCP发送消息框", array type (2D Dbl)=u8[] []) -> (array=w513:u8[])
                          n273 = Byte Array To String(unsigned byte array=w513) -> (string=w509:string)
                          n274 = Concatenate Strings(w509, "\r\n") -> (w508:string)
                        }
                      }
                    }
                  }
                  n275 = TCP Write(connection ID=w493, data in=w490, error in (no error)=w492) -> (connection ID out=w488:refnum<k5>, error out=w489:errorcluster)  [unwired: 1 in, 1 out]
                }
              }
            }
          }
          n276 = local read "开启监听"() -> (w478:bool)
          n277 = Exclusive Or(1:TRUE ("y"), 2:w478) -> (0:w476:bool)
        }
        n278 = while {
          tunnel: [w523] -> w469
          tunnel: [w522] -> w475
          tunnel: w472 -> [w520]
          tunnel: w471 -> [w521]
          stop <- w516 stop-if-true
          n279 = case shown="真" "TCP HEX" {
            tunnel: [w538 w546] -> w523
            tunnel: [w539 w545] -> w522
            tunnel: w521 -> [w540 w544]
            tunnel: w520 -> [w541 w543]
            frame True {
              w526 = 2 ("y")
              n280 = TCP Read(connection ID=w541, bytes to read=1 ("读取的字节"), error in (no error)=w540, 7:T1."CRLF" ("模式（标准）")) -> (connection ID out=w539:refnum<k5>, data out=w537:string, error out=w538:errorcluster)  [unwired: 1 in]
              n281 = property on="TCP接收信息框" class="Str"("Text.Scroll Position"=inf) -> ()  [unwired: 2 in, 2 out]
              n282 = String To Byte Array(string=w537) -> (unsigned byte array=w536:u8[])
              n283 = call <vilib>:"Space Constant.vi"() -> ("String"=w534:string)
              n284 = call <vilib>:"Space Constant.vi"() -> ("String"=w530:string)
              n285 = Array To Spreadsheet String(delimiter (Tab)=w534, array=w536, 3:"%x" ("格式字符串")) -> (spreadsheet string=w529:string)
              n286 = String Length(string=w529) -> (length=w528:i32)
              n287 = Subtract(x=w528, y=w526) -> (x-y=w527:i32)
              n288 = local read "TCP接收信息框"() -> (w532:string)
              n289 = Replace Substring(2:w526, 3:w527, 4:w530, 5:w529) -> (1:w525:string)  [unwired: 1 out]
              n290 = Concatenate Strings(w532, w525) -> (w533:string)
              n291 = local write "TCP接收信息框"(w533) -> ()
            }
            frame False {
              n292 = property on="TCP接收信息框" class="Str"("Text.Scroll Position"=inf) -> ()  [unwired: 2 in, 2 out]
              n293 = local read "TCP接收信息框"() -> (w552:string)
              n294 = TCP Read(connection ID=w543, bytes to read=1 ("读取的字节"), error in (no error)=w544, 7:T1."CRLF" ("模式（标准）")) -> (connection ID out=w545:refnum<k5>, data out=w551:string, error out=w546:errorcluster)  [unwired: 1 in]
              n295 = Concatenate Strings(w552, w551) -> (→"TCP接收信息框":string)
            }
          }
          n296 = local read "开启监听"() -> (w518:bool)
          n297 = Exclusive Or(1:TRUE ("y"), 2:w518) -> (0:w516:bool)
        }
        n298 = TCP Close Connection(connection ID=w475, error in (no error)=w469) -> ()  [unwired: 1 in, 2 out]
        n299 = call <vilib>:"Clear Errors.vi"("error in (no error)"=w469, "specific error code to clear (0: all)"=w467) -> ()  [unwired: 4 in, 2 out]
        n300 = call <vilib>:"Clear Errors.vi"("error in (no error)"=w468, "specific error code to clear (0: all)"=w467) -> ()  [unwired: 4 in, 2 out]
        n301 = TCP Close Connection(connection ID=w470, error in (no error)=w468) -> ()  [unwired: 1 in, 2 out]
      }
    }
  }
  n302 = VISA Close(VISA resource name=w5, error in (no error)=w8) -> ()  [unwired: 1 out]
